vi "Automatic Frequency Linearization.vi"() -> ()   [LabVIEW 2014]
panel:
  in  "StopValue":dbl
  in  "stop":bool
  out "Mean  FREQUENCY Curve Falling":dbl[](graph)
  out "Mean FREQUENCY Curve Rising":dbl[](graph)
  out "Current Skew Tri":dbl[](graph)
  out "Current mul factor":dbl
  out "Current iteration (Countdown)":dbl
  out "rising<= 1%":bool
  out "falling<= 1%":bool
  in  "DeltaFactor":dbl=0.01
  in  "Initial Factor Mul":dbl=0.5
  out "2) Rising StdDev % Graph":cluster{dbl[], dbl[]}(graph)
  out "1) Falling StdDev % Graph":cluster{dbl[], dbl[]}(graph)
  out "2) Rising Std Dev %":dbl
  out "1) Falling Std Dev %":dbl
  out "2) Rising Signal (Last)":dbl[](graph)
  out "1) Falling Signal (Last)":dbl[](graph)
  in  "#Mesuraments":i32=20
  # "OFFLINE SETUP"
  # "CURRENT ITERATION"
  # "Numero di misurazioni\n su cui mediare"
  # "Fattore moltiplicativo\nIniziale"
  # "Passo del fattore\nmoltiplicativo"
  # "Optimal Factor Rising: 0.33    with Falling curve: 0.294"
  # "Optimal Factor Falling: 0.22/0.23"
  # "Raccomended:\n#Mean: 20\nInitial: 0,3\nStep: 0,01"
  # "%"
  # "%"
  # "FINAL RESULTS"
  # "Andamento della deviazione standard percentuale in funzione del fattore moltiplicativo"
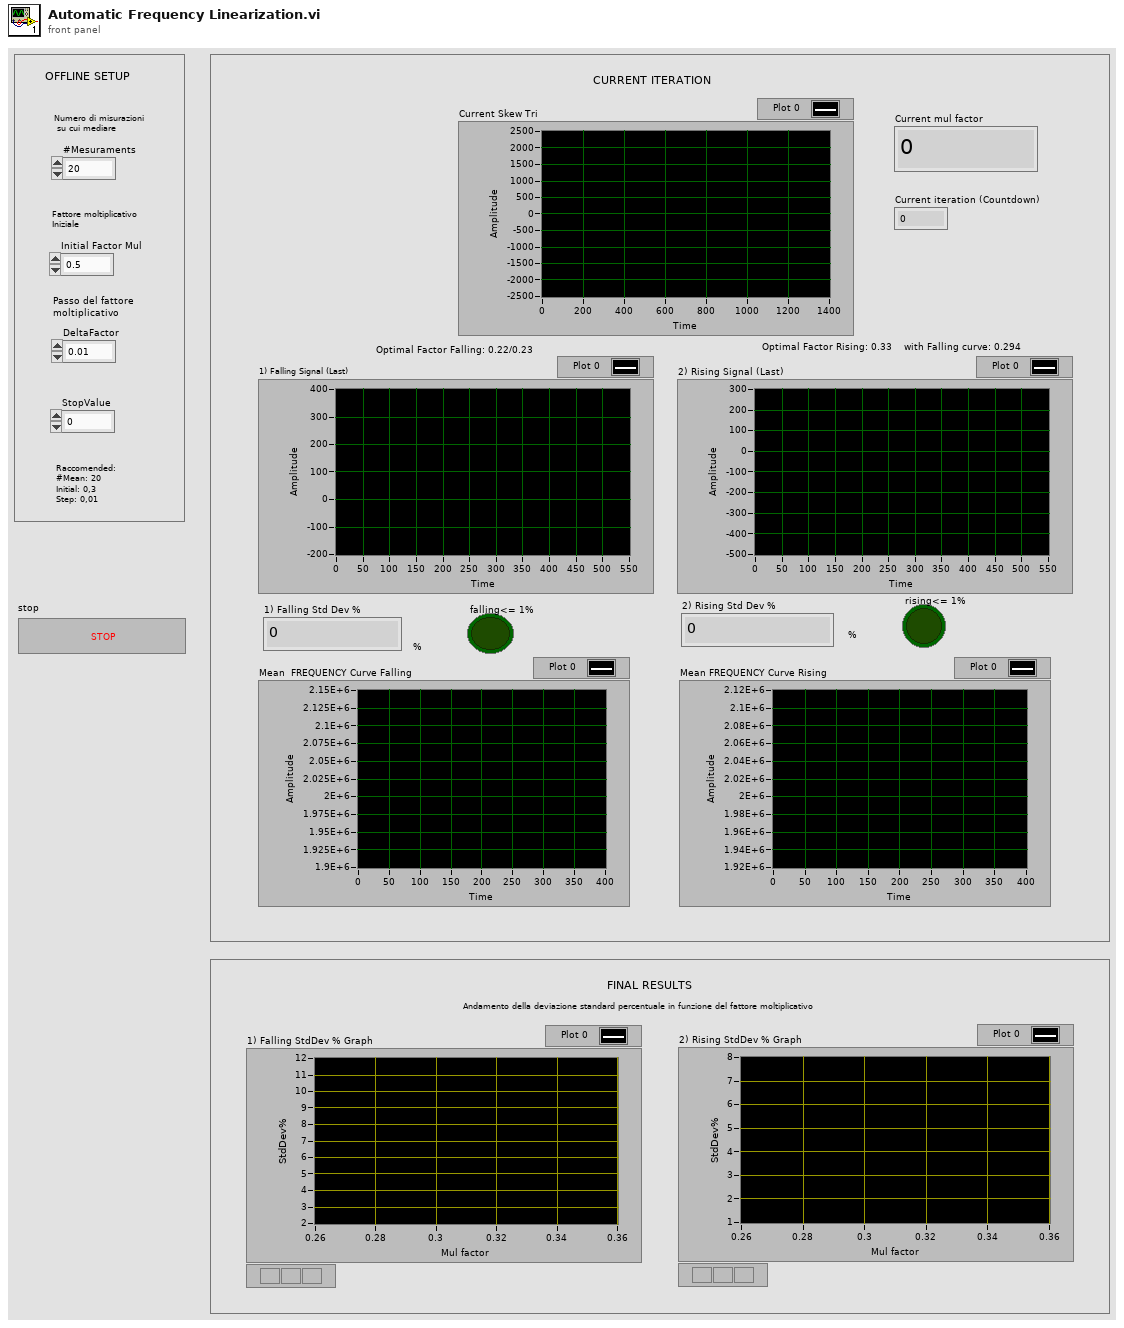
[diagram p1: front panel]
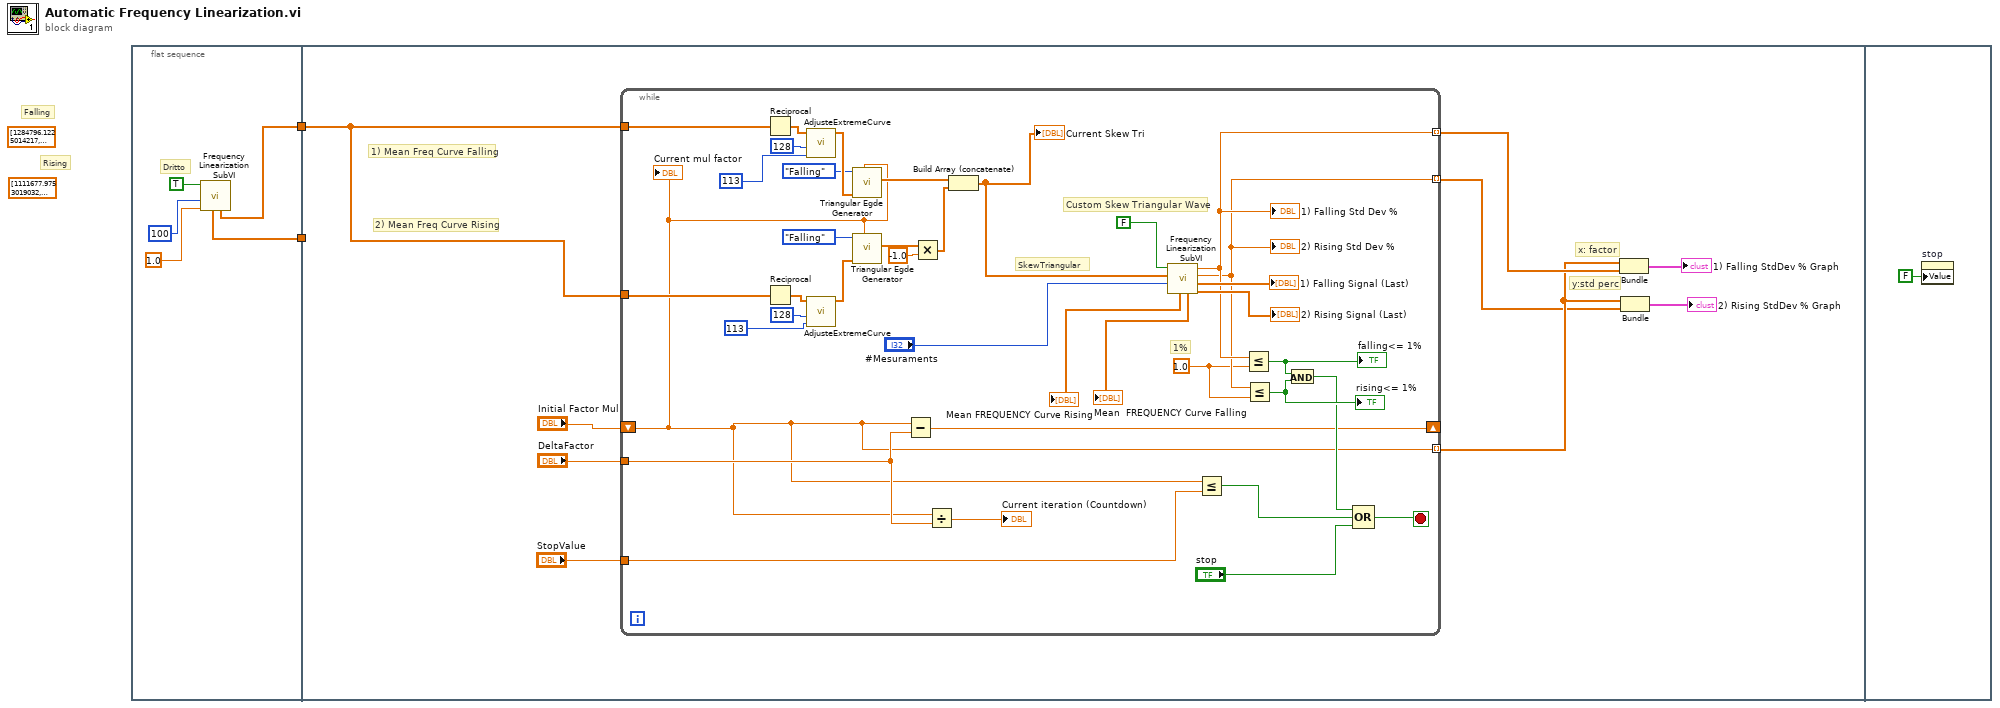
[diagram p0: block diagram]
diagram:
  (unwired) dbl[] [1284796.1225014217, 1294107.7987199828, 1303745.0098122759, 1310174.1525820007, 1321007.4949358704, 1331266.171826723, 1340421.5960605256, 1347335.8699514961, 1355371.0637180319, 1362899.6091552188, 1369064.2510553782, 1375324.267925689, 1381671.7114464506, 1388095.7102428216, 1394583.1783171922, 1401119.4925036891, 1407689.4935558552, 1414279.3095683786, 1420877.9730196733, 1427477.7482344015, 1434073.5994277853, 1440662.3820554372, 1447241.7381296123, 1454665.9396385304, 1461145.6616659332, 1468607.123461634, 1475907.2789256435, 1482164.4311400491, 1490680.0141473096, 1499634.011576698, 1505455.6984635997, 1513903.1691790659, 1520968.430435831, 1529853.6870611566, 1539016.6831225976, 1550214.4221631626, 1557222.2596074783, 1567842.8170041486, 1576844.7930965954, 1584799.5366042946, 1592515.3345920537, 1600521.8957773142, 1610579.6946919337, 1618188.301714767, 1624451.8674566182, 1630858.9839059033, 1636119.1543515318, 1643597.063353953, 1648999.8443721235, 1654415.7035595593, 1659841.967615204, 1665885.1507876618, 1671368.5941808412, 1676844.1977378346, 1682303.873760102, 1687739.7515589865, 1693145.4553829404, 1698517.4085751562, 1703855.6016353904, 1709163.488948023, 1714446.8228577834, 1719711.493605011, 1724961.0845179735, 1730195.5348681135, 1735411.2201350871, 1740601.5971745611, 1745758.223187119, 1750872.5240667071, 1755937.5728629916, 1760949.31592121, 1765907.2514703749, 1770814.1577267686, 1776696.8606506076, 1781464.7975645186, 1786199.2156875923, 1790902.646740379, 1796519.1813009335, 1801708.1327623287, 1806853.8212386095, 1811356.6519549456, 1817147.878317621, 1821839.1344470838, 1826640.357393866, 1831959.6756015208, 1836571.9050816444, 1841767.23541417, 1847267.099846194, 1852939.8822536138, 1857627.6008608802, 1863499.69504039, 1868983.0459327814, 1874469.997387419, 1880149.1058005956, 1886456.1414375356, 1892377.116971627, 1898693.3277808323, 1903709.1374254432, 1908567.4527627965, 1913507.536131368, 1918482.4274221116, 1922679.4877879873, 1927109.1926845738, 1931865.936337121, 1936619.651214964, 1940541.1064024847, 1944457.7593437028, 1949305.023085125, 1953269.599495912, 1957220.6869914997, 1961800.2766758106, 1965723.8227072882, 1969615.0884177368, 1973471.5713236644, 1977293.5687343879, 1981084.6101625597, 1984850.739743371, 1988598.6968028292, 1992333.4633422785, 1996056.2750668826, 1999764.9078377516, 2003455.4969125378, 2007124.410604366, 2010770.206769693, 2014395.1475538525, 2018004.721953882, 2021605.1847636478, 2025200.9927104136, 2028793.613267417, 2032381.0624314705, 2035958.34281758, 2039519.6050135384, 2043060.943208106, 2046582.2483926967, 2050087.1031018472, 2053581.1632508596, 2057070.0282333065, 2060556.8196814083, 2064040.6394989977, 2067517.2075212854, 2070980.593035177, 2074424.8096369302, 2077845.156969661, 2081238.9233311191, 2084605.4911244228, 2088080.7207846858, 2091387.3259896142, 2094675.7838649538, 2097947.3264351254, 2101201.0832521413, 2104434.746222321, 2107645.6971964967, 2110832.3759229127, 2113995.4450913155, 2117137.817565047, 2120263.3910007, 2123718.3858808614, 2126975.5149182007, 2130621.2944829953, 2133578.8209881335, 2136678.5409494443, 2139735.460015835, 2142702.9743946767, 2146306.9436483094, 2149862.718588536, 2152999.0998194064, 2156091.497046698, 2159317.54521168, 2162006.3248660546, 2166865.8796383115, 2169677.97115338, 2172556.901358816, 2177113.284060673, 2180213.8539566174, 2183751.81677155, 2186715.59177596, 2189661.524360636, 2193357.8909541154, 2196736.1623947285, 2199507.123696312, 2202962.338836369, 2205970.1168696983, 2209371.9781521284, 2211552.0679771663, 2214236.8325021397, 2217016.601835507, 2220368.193650237, 2223432.4495542576, 2226043.869256761, 2228449.4938743813, 2231114.1947228415, 2233631.2545425696, 2236337.2814795286, 2239020.2563699232, 2241555.732577774, 2244626.6372566265, 2247325.914570994, 2249801.181413759, 2253426.868824545, 2255921.9715584223, 2258085.0712267817, 2260573.779686374, 2263057.903219097, 2266098.1001831144, 2268578.502537367, 2271055.47575304, 2274006.997136441, 2276491.221797948, 2278976.117241898, 2281466.7826434774, 2283967.96994154, 2286481.962726374, 2289007.561515149, 2291540.798392755, 2294076.820964208, 2296611.4330864507, 2299141.656239755, 2301665.7324047913, 2304182.8955696416, 2306693.1817105226, 2309197.0804978115, 2311694.4899604847, 2314183.7397563076, 2316661.9511477984, 2319126.723647868, 2321577.884558988, 2324017.735471777, 2326449.5389530268, 2328875.376030322, 2331294.8487004116, 2333704.9029559586, 2336100.725482478, 2338477.73857972, 2340832.9859676417, 2343165.0250034924, 2345473.5779788373, 2347759.2048304896, 2350022.4669374707, 2352262.8016105928, 2354478.2083023726, 2356665.900779324, 2358823.1829853584, 2360948.402080695, 2363041.9752920126, 2365106.550371168, 2367145.674188815, 2369161.667724184, 2371154.1965097953, 2373120.7837049845, 2375058.1555777327, 2376963.6759592886, 2378837.0223877267, 2380680.5326322145, 2382497.295352574, 2384288.9227429326, 2386239.9643591116, 2387951.4295912273, 2389635.7334956587, 2391291.0888577714, 2392916.328786578, 2394511.3251612023, 2396077.2488878486, 2397616.245853075, 2399130.691921395, 2400622.2845292846, 2402091.2616443355, 2403536.7116874475, 2404958.6947879326, 2406359.715835251, 2407743.8597365757, 2409115.0848977403, 2410476.07655086, 2411828.0382462633, 2413171.4365479248, 2414082.6639564345, 2415372.109253754, 2416657.826946633, 2417941.751744223, 2419225.817120007, 2420512.4789449098, 2421804.2327939277, 2423102.7583092935, 2424408.657594866, 2425722.2911311267, 2427045.4440690516, 2428382.0095616807, 2429736.5993662095, 2431112.510123017, 2432592.3095966694, 2434003.155028903, 2435435.223106938, 2436888.1567866374, 2438361.6793758767, 2440037.5920760646, 2441513.299017333, 2443008.2079034336, 2444522.8241073433, 2446216.834038796, 2447681.1053035883, 2449243.354007954, 2450949.8084933283, 2452552.6845717393, 2454183.570787015, 2456630.664047362, 2458284.9942586627, 2460178.4779965105, 2461572.505250558, 2463848.358183508, 2465664.127487748, 2467288.396246923, 2468931.504028505, 2470161.635017583, 2471936.3756099753, 2473568.58590929, 2475016.3362461333, 2476424.2598212217, 2477833.5758932102, 2480127.4867510335, 2481743.9551331946, 2484242.010379677, 2485657.8344102935, 2487085.736879674, 2489127.3980101934, 2490690.6577383745, 2492211.8838634794, 2493176.2609678074, 2494823.7453838624, 2496163.3126188596, 2497893.310215999, 2499368.4262579726, 2500979.603476495, 2502655.391472255, 2504835.5483735455, 2506423.966758712, 2507728.4580071266, 2509516.839256799, 2510729.40818521, 2512309.0676383204, 2514632.963503338, 2516241.884496811, 2517531.0923509104, 2518945.2829947025, 2521016.7808592985, 2522311.6638790877, 2524009.0228848453, 2525806.038975564, 2527118.5927077625, 2528221.572172253, 2529883.1168161053, 2530799.5559831257, 2532089.7984877755, 2533429.806421817, 2534684.4436777933, 2535947.602398312, 2537316.749515253, 2538784.1414706847, 2540089.857341136, 2541854.3460449977, 2543599.2117023272, 2544902.048730936, 2546199.0341286133, 2547489.0490999846, 2548771.8061365387, 2550047.744776987, 2551169.0058938884, 2552880.632386139, 2554306.07208447, 2555566.2650138717, 2558207.246486741, 2559762.791616098, 2561148.405324582, 2562356.126305806, 2564286.770006348, 2565522.1440156205, 2566866.175670722, 2568171.5688289325, 2569330.7816873007, 2570463.4191790186, 2571569.043973086, 2572648.641950922, 2573705.249646773, 2574743.3689784, 2575767.5546550304, 2576781.2584241573, 2577786.352045087] ("1) Mean Freq Curve Falling")
  (unwired) dbl[] [1111677.9753019032, 1117543.1447773844, 1124727.071271594, 1130759.2368636343, 1139900.9987218028, 1147005.724525075, 1155597.805965007, 1161653.374065326, 1175017.7759895455, 1184554.3352683126, 1198642.8299017954, 1209710.0333819909, 1220635.0664652071, 1226484.7218799912, 1239228.804919277, 1251542.9142337078, 1261646.6139546419, 1274582.176220145, 1285436.5489759166, 1296816.369294055, 1306515.9760767864, 1314666.8762996064, 1324981.646261902, 1334658.0888899087, 1343132.6189077713, 1349098.9058813928, 1355074.8712651432, 1361052.6107200729, 1367024.6270163925, 1372985.1513636126, 1378930.872879021, 1384861.1503988027, 1390778.0276034328, 1396685.6748278143, 1402588.9011085096, 1408491.456899597, 1414394.8988214084, 1420298.0445305281, 1426196.931912433, 1432085.2034800425, 1437955.0485002107, 1443798.393505134, 1450256.918642635, 1455942.696976346, 1461590.0930875582, 1467201.08557465, 1473277.3769945034, 1478787.2520329228, 1486500.7495878495, 1492491.1652184343, 1497811.278392427, 1503130.7312790786, 1511258.741224468, 1518371.941122686, 1525976.391146262, 1535560.057102009, 1545227.8649395378, 1554643.9601199678, 1561734.137510287, 1567652.326824544, 1573363.3384242547, 1580371.4268145494, 1589269.3702707214, 1599544.6527499703, 1606524.9429361785, 1613244.9205027358, 1619570.8592119175, 1626167.1449764848, 1631910.8176346058, 1638084.9774862805, 1643579.6051365405, 1649651.596378431, 1654735.1400781763, 1660662.0324426997, 1665798.7946457735, 1670947.7823896396, 1676112.9396798953, 1681293.4983906904, 1686484.2602242208, 1691676.8939355335, 1696861.9618521526, 1702031.253903078, 1707179.5063695384, 1712305.1662937002, 1717410.2409879356, 1722499.1364517482, 1727576.729324952, 1732646.5184208567, 1737709.3846412706, 1742763.2984129312, 1747803.7647843692, 1752824.8106602966, 1757820.876302829, 1762788.918364598, 1767729.303416593, 1772645.2806915073, 1777541.7086792772, 1782423.599880446, 1787769.673996657, 1793098.2752046043, 1799032.6873749204, 1803743.0682482957, 1808688.8606219003, 1814111.1746080806, 1818833.8038602145, 1824218.044046183, 1828738.2588971546, 1834747.0545098886, 1841687.0094862306, 1848274.3160562834, 1853425.3967999006, 1858462.4230257096, 1865975.304215294, 1872323.7778459906, 1879829.7369455763, 1886255.2182835734, 1890827.261980319, 1895892.0242774424, 1902974.8929223255, 1908649.6601406157, 1915330.5466930955, 1919469.800142402, 1925861.342977329, 1931524.1005310323, 1935680.7737204009, 1940609.151881379, 1945339.6191252808, 1949855.3037516465, 1954022.7359062806, 1958175.156107716, 1962688.9725794748, 1966834.9088139278, 1970974.19436239, 1975697.3367558725, 1979845.3153871722, 1983974.0204327945, 1988080.2990186054, 1992164.2309316027, 1996228.6063043787, 2000277.502570961, 2004314.3954349258, 2008340.4389004973, 2012353.7479727361, 2016350.1640284169, 2020324.679919784, 2024272.5142174596, 2028190.4248440834, 2032078.2956945268, 2035939.644973722, 2039780.4922710317, 2043606.9332988367, 2047422.908713295, 2051229.3077925856, 2055024.141795437, 2058803.6897034254, 2062564.3266697822, 2066304.3171184964, 2070025.204635398, 2073732.0447149184, 2077432.024213566, 2081132.2617511034, 2085298.621896397, 2088977.5375496647, 2092659.6763426436, 2096341.2492383083, 2100019.5102272155, 2103694.7155473772, 2107369.9286785023, 2111611.867390658, 2115729.0796630206, 2119852.470853293, 2123467.897868767, 2127905.307749301, 2131489.0985475457, 2135542.9497605534, 2139319.351740196, 2143611.943816123, 2147452.633133921, 2151141.1699249553, 2155287.4797924925, 2159580.4500603555, 2163104.3948940937, 2166878.958964213, 2171406.1162917768, 2176234.501059857, 2180462.7042502193, 2186243.4827238084, 2190022.378374309, 2194567.7863056003, 2199534.3635077667, 2203861.798662165, 2208515.375563887, 2212049.8622649307, 2216336.364381327, 2219871.6096689953, 2223163.156841111, 2226423.4079460637, 2230578.1181568145, 2234538.464659099, 2238593.6655228357, 2242063.6372863413, 2245399.565919357, 2248782.5576294125, 2252497.8162754457, 2255723.1459333394, 2258947.3995064646, 2262172.1814569146, 2265397.5643387083, 2268621.650488728, 2272182.314735969, 2275412.304717649, 2278955.5911732004, 2282170.3148253304, 2285370.4102494516, 2288559.9049064214, 2291744.208951241, 2294927.5919124396, 2298111.2569676577, 2301922.2440816606, 2305133.6720987437, 2308334.1866843887, 2311524.857056277, 2314709.3122709147, 2317891.745493507, 2321074.9496455877, 2324258.7850316493, 2327439.9676925107, 2330613.5021329997, 2333774.922256018, 2336922.391707122, 2340057.7161509986, 2343185.339063086, 2346309.5390550303, 2349432.115077642, 2352552.263973642, 2355667.5968150655, 2358775.2763190563, 2361873.2891140147, 2364961.975310351, 2368044.83411824, 2371127.392140788, 2374214.772380495, 2377309.6262211185, 2380411.452017836, 2383517.416752593, 2386624.547798929, 2389731.963716068, 2392841.471619131, 2395956.22678397, 2399078.6025783936, 2402209.054938916, 2405346.2279427783, 2408487.8152081617, 2411631.5597667857, 2414775.573352531, 2417926.963015192, 2421053.5337855695, 2424183.725236519, 2427319.6977999173, 2430461.617861762, 2433606.4857367193, 2436865.3295776444, 2440461.9281352838, 2443668.7948092353, 2446416.1420945805, 2449410.83597939, 2452372.7406688067, 2455361.7211039755, 2458726.078587466, 2461703.7860250506, 2464918.529947554, 2468403.9370960705, 2471883.210584818, 2474845.3964347276, 2478549.8873876333, 2481597.6511591743, 2484974.3582069697, 2487508.413522569, 2491204.290929187, 2494296.47608529, 2497884.7618336543, 2500377.8385557854, 2503380.4497023877, 2505895.4122516173, 2508623.4130788953, 2511236.9306225497, 2513885.7596208784, 2516788.7099948106, 2518973.653531057, 2521682.8080157526, 2523947.8732564123, 2527088.896197209, 2529678.699091686, 2532246.637863351, 2535068.548296424, 2537665.22096253, 2539840.737862212, 2542583.5429503457, 2544895.037672506, 2547109.1212503216, 2549492.815290109, 2551724.051181589, 2554190.7292130576, 2556440.7182187494, 2558969.0706954645, 2561386.315215632, 2564072.761457738, 2566682.4907546053, 2569093.976621355, 2571521.2130877757, 2573963.361788066, 2576421.9006172004, 2578899.6402907907, 2581398.8577477247, 2583919.6417094106, 2586459.446920175, 2589014.4418694596, 2591581.1394325625, 2594157.428460757, 2596743.502536236, 2599342.117480276, 2601957.254014361, 2604591.6693875585, 2607245.1424855883, 2609914.642877777, 2612596.398246293, 2615288.2478070064, 2617990.2382559944, 2620703.403495802, 2623428.04275305, 2626162.3180289413, 2628902.3527476224, 2631643.861737056, 2634383.3932900704, 2637119.2478786297, 2639852.1813324727, 2642584.125598411, 2645315.5497193234, 2648044.2823686963, 2650766.3203635095, 2653477.4540122817, 2656175.271021147, 2658860.524969149, 2661536.2929979516, 2664205.570514177, 2666869.43481786, 2669526.6226534448, 2672174.2393878074, 2674809.4740124578, 2677431.685642747, 2680042.6550569087, 2682644.3580223606, 2685236.7148642833, 2687817.204705562, 2690382.002405132, 2692927.3120981795, 2695450.756861085, 2697952.914930008, 2700437.241443272, 2702907.9023478995, 2705367.553726213, 2707816.2586694118, 2710252.0953420424, 2712673.419901639, 2715080.622190063, 2717475.41680173, 2719858.803281426, 2722229.9796343716, 2724586.533823991, 2726925.7222361835, 2729245.7377309934, 2731545.975438041, 2733827.6130194296, 2736094.288495403, 2738351.057123957, 2740601.8310580896, 2742847.545018403, 2745087.399218133, 2747321.4806488585, 2749551.2825875836, 2751778.138271394, 2754001.674772157, 2756230.9359481973, 2758405.7222731416] ("2) Mean Freq Curve Rising")
  # "Rising"
  # "Falling"
  n1 = flat-sequence {
    tunnel: [w4] -> w2
    tunnel: [w3] -> w1
    tunnel: w2 -> [w8]
    tunnel: w1 -> [_]
    frame #0 {
      # "Dritto"
      n2 = call "Frequency Linearization SubVI.vi"("Scale factor"=1.0, "#Medie"=100, "Triangolo dritto"=TRUE) -> ("Last Mean Freq Curve Falling"=w4:dbl[], "Last Mean Freq Curve Rising"=w3:dbl[])  [unwired: 3 in, 4 out]
    }
    frame #1 {
      # "2) Mean Freq Curve Rising"
      # "1) Mean Freq Curve Falling"
      # "y:std perc"
      # "x: factor"
      n3 = while {
        tunnel: [w49] -> w14 mode=indexing
        tunnel: [w48] -> w10 mode=indexing
        shift-right: [w21] -> _
        shift-left: "Initial Factor Mul" -> [w17]
        tunnel: "DeltaFactor" -> [w19]
        tunnel: w8 -> [w34]
        tunnel: w8 -> [w32]
        tunnel: [w17] -> w11 mode=indexing
        tunnel: "StopValue" -> [w18]
        stop <- w24 stop-if-true
        w47 = 1.0 ("y")
        # "SkewTriangular"
        # "1%"
        # "Custom Skew Triangular Wave"
        n4 = Reciprocal(x=w34) -> (1/x=w33:dbl[])
        n5 = Reciprocal(x=w32) -> (1/x=w45:dbl[])
        n6 = call "AdjusteExtremeCurve.vi"("Init Bins Discarded"=u32 113, "FFT Size Window"=128, "Freq sample"=w33) -> ("Extended Freq Sample"=w38:dbl[])  [unwired: 8 in]
        n7 = call "AdjusteExtremeCurve.vi"("Init Bins Discarded"=u32 113, "FFT Size Window"=128, "Freq sample"=w45) -> ("Extended Freq Sample"=w39:dbl[])  [unwired: 8 in]
        n8 = call "Triangular Egde Generator.vi"("fattore"=w17, "Sample values"=w38, "Triangular edge"=enum16{"Rising", "Falling"}."Falling") -> ("Skew Triangular"=w37:dbl[])  [unwired: 8 in]
        n9 = call "Triangular Egde Generator.vi"("fattore"=w17, "Sample values"=w39, "Triangular edge"=enum16{"Rising", "Falling"}."Falling") -> ("Skew Triangular"=w41:dbl[])  [unwired: 8 in]
        n10 = Subtract(x=w17, y=w19) -> (x-y=w21:dbl)
        n11 = Multiply(x=w41, y=-1.0) -> (x*y=w42:dbl[])
        n12 = Divide(x=w17, y=w19) -> (x/y=→"Current iteration (Countdown)":dbl)
        n13 = Build Array (concatenate)(w37, w42) -> (w31:dbl[])
        "Current Skew Tri" <- w31
        n14 = call "Frequency Linearization SubVI.vi"("#Medie"="#Mesuraments", "Sketri Input"=w31, "Triangolo dritto"=FALSE) -> ("Second Signal (Last)"=→"2) Rising Signal (Last)":dbl[], "First Signal (Last)"=→"1) Falling Signal (Last)":dbl[], "Rising Std Dev %"=w48:dbl, "Falling Std Dev %"=w49:dbl, "Last Mean Freq Curve Falling"=→"Mean  FREQUENCY Curve Falling":dbl[], "Last Mean Freq Curve Rising"=→"Mean FREQUENCY Curve Rising":dbl[])  [unwired: 3 in]
        "1) Falling Std Dev %" <- w49
        "2) Rising Std Dev %" <- w48
        n15 = Less Or Equal?(x=w17, y=w18) -> (x <= y?=w20:bool)
        n16 = Less Or Equal?(x=w49, y=w47) -> (x <= y?=w50:bool)
        "falling<= 1%" <- w50
        n17 = Less Or Equal?(x=w48, y=w47) -> (x <= y?=w46:bool)
        "rising<= 1%" <- w46
        n18 = And(x=w50, y=w46) -> (x .and. y?=w23:bool)
        n19 = Compound Arithmetic op=OR(w23, w20, "stop") -> (w24:bool)
        "Current mul factor" <- w17
      }
      n20 = Bundle(w11, w14) -> (→"1) Falling StdDev % Graph":cluster{dbl[], dbl[]})  [unwired: 1 in]
      n21 = Bundle(w11, w10) -> (→"2) Rising StdDev % Graph":cluster{dbl[], dbl[]})  [unwired: 1 in]
    }
    frame #2 {
      n22 = property on="stop" class="Bool (strict)"("Value"=FALSE ("stop")) -> ()  [unwired: 2 in, 2 out]
    }
  }
